vi "save_bin2t.vi"(0 "Cluster":T1, 1 "Dev_Gr":cluster{"DevNo":i32, "Group":string}[](array[cluster]), 2 "Data Directory":path, 3 "Save2disk":refnum<vi>) -> ()   [LabVIEW 2010]
uses:
  lib/Global 2.vi
  lib/to_utc.vi
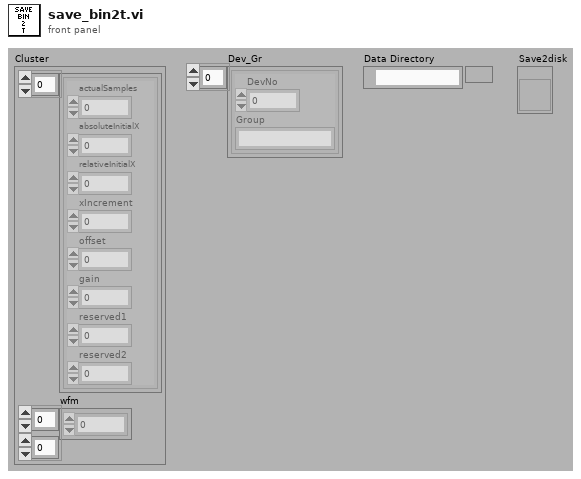
[diagram p1: front panel]
types:
  T1 = cluster{cluster{"actualSamples":i32, "absoluteInitialX":dbl, "relativeInitialX":dbl, "xIncrement":dbl, "offset":dbl, "gain":dbl, "reserved1":dbl, "reserved2":dbl}[], "wfm":i16[][]}
  T2 = cluster{"name":enum16{"sync", "phase_a", "phase_b", "phase_c", "ground"}, "num":i32, "Numeric":i32}[]
  T3 = cluster{"actualSamples":i32, "absoluteInitialX":dbl, "relativeInitialX":dbl, "xIncrement":dbl, "offset":dbl, "gain":dbl, "reserved1":dbl, "reserved2":dbl}[]
  T4 = cluster{cluster{"actualSamples":i32, "absoluteInitialX":dbl, "relativeInitialX":dbl, "xIncrement":dbl, "offset":dbl, "gain":dbl, "reserved1":dbl, "reserved2":dbl}[], i16[][]}
  T5 = cluster{"actualSamples":i32, "absoluteInitialX":dbl, "relativeInitialX":dbl, "xIncrement":dbl, "offset":dbl, "gain":dbl, "reserved1":dbl, "reserved2":dbl}
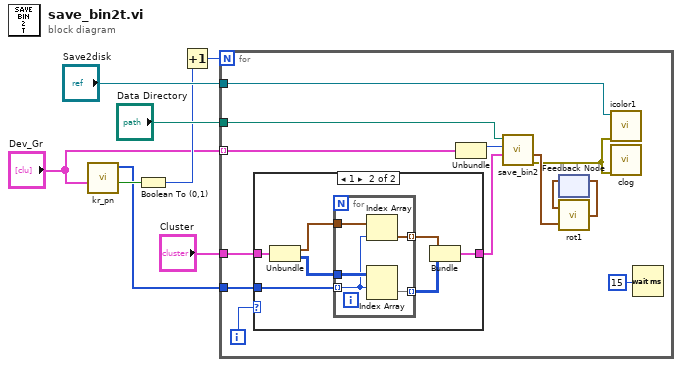
[diagram p0: block diagram]
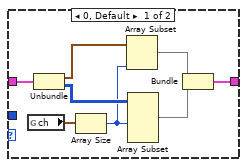
[diagram p2: hidden frame]
diagram:
  n1 = call "kr_pn.vi"("Dev_Gr"="Dev_Gr") -> ("x = y?"=w6:bool, "Array"=w1:i32[])  [unwired: 3 in, 2 out]
  n2 = Boolean To (0,1)(Boolean=w6) -> (0, 1=w5:i16)
  n3 = Increment(x=w5) -> (x+1=w4:i16)
  n4 = for {
    N: w4 -> [_]
    tunnel: "Data Directory" -> [w21]
    tunnel: "Save2disk" -> [w20]
    tunnel: "Cluster" -> [w12]
    tunnel: "Dev_Gr" -> [w15] mode=indexing
    tunnel: w1 -> [w10]
    i -> [w9]
    n5 = case shown="1" w9 {
      tunnel: w10 -> [_ w36]
      tunnel: w12 -> [w29 w35]
      tunnel: [w28 w30] -> w11
      frame 0, Default {
        n6 = global read "Global 2.vi" "ch"() -> (w22:T2)
        n7 = Unbundle(w29) -> (w27:T3, "wfm"=w26:i16[][])
        n8 = Array Size(array=w22) -> (size(s)=w23:i32)
        n9 = Array Subset(array=w27, length=w23) -> (w25:T3)  [unwired: 1 in]
        n10 = Array Subset(array=w26, length (row)=w23) -> (w24:i16[][])  [unwired: 3 in]
        n11 = Bundle(w25, w24) -> (w28:T4)  [unwired: 1 in]
      }
      frame 1 {
        n12 = Unbundle(w35) -> (w33:T3, "wfm"=w34:i16[][])
        n13 = for {
          tunnel: w36 -> [w38] mode=indexing
          tunnel: [w41] -> w31 mode=indexing
          tunnel: w34 -> [w40]
          tunnel: w33 -> [w39]
          tunnel: [w37] -> w32 mode=indexing
          n14 = Index Array(array=w39, index=w38) -> (element=w37:T5)
          n15 = Index Array(array=w40, index (row)=w38) -> (element=w41:i16[])  [unwired: 1 in]
        }
        n16 = Bundle(w32, "wfm"=w31) -> (w30:T1)  [unwired: 1 in]
      }
    }
    n17 = Unbundle(w15) -> ("DevNo"=w14:i32)  [unwired: 1 out]
    n18 = call "save_bin2.vi"("xz"=w11, "DevNo"=w14, "start path"=w21) -> ("error out"=w16:errorcluster, "timestamp"=w17:timestamp)  [unwired: 2 in, 1 out]
    n19 = feedback #1() -> (w18:timestamp[])  [unwired: 1 in]
    n20 = call "rot1.vi"("t0"=w17, "input"=w18) -> ("output array"=w19:timestamp[])
    n21 = feedback-in #1(w19) -> ()
    n22 = call "icolor1.vi"("error in (no error)"=w16, "Bool Refnum"=w20) -> ()  [unwired: 6 in]
    n23 = call "clog.vi"("error"=w16) -> ()  [unwired: 7 in]
    n24 = Wait (ms)(milliseconds to wait=u32 15) -> ()  [unwired: 1 out]
  }
